vi "7-29-19 Decreasing.vi"() -> ()   [LabVIEW 2016]
uses:
  <userlib>/Levylab/LV to ITX/LVtoITX.lvclass
  <vilib>/Analysis/NI_AALPro.lvlib
panel:
  out "dG/dt Vs Temp Normalized":cluster{"Data":dbl[], "Data":dbl[]}[](graph)
  out "Slopes":cluster{dbl[], dbl[]}
  out "G Vs Time Fitted":cluster{"Data":dbl[], "Data":dbl[]}[](graph)
  out "Wavenames":string[](array[string])
  out "G Vs Time":cluster{"Data":dbl[], "Data":dbl[]}[](graph)
  out "Data":dbl[][](array[numeric])
  in  "File Path":path=path "G:/My Drive/Data/7-30 Decreasing SA03083.dat"
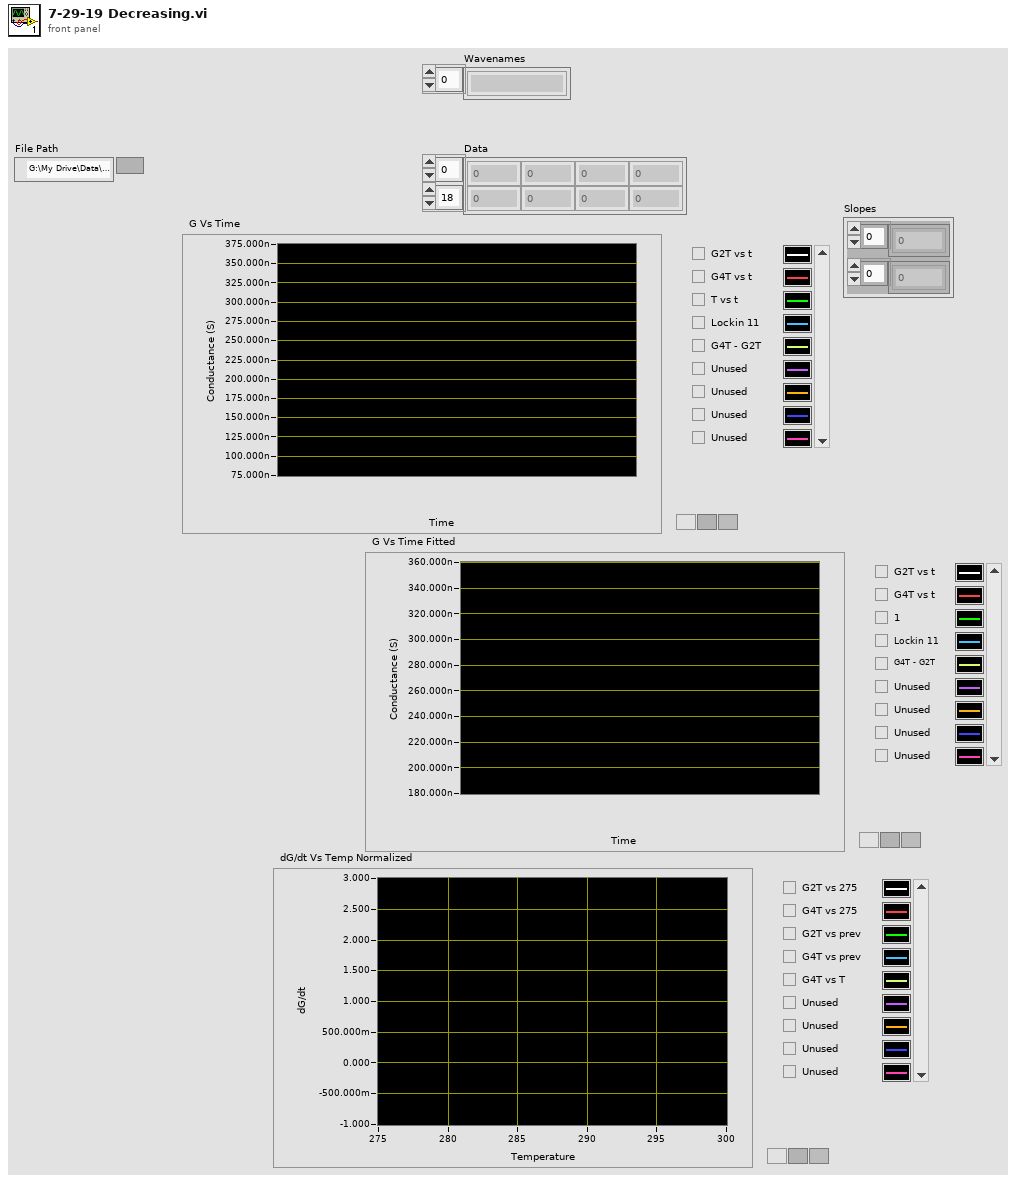
[diagram p1: front panel]
types:
  T1 = cluster{"slope min":dbl, "slope max":dbl, "intercept min":dbl, "intercept max":dbl}
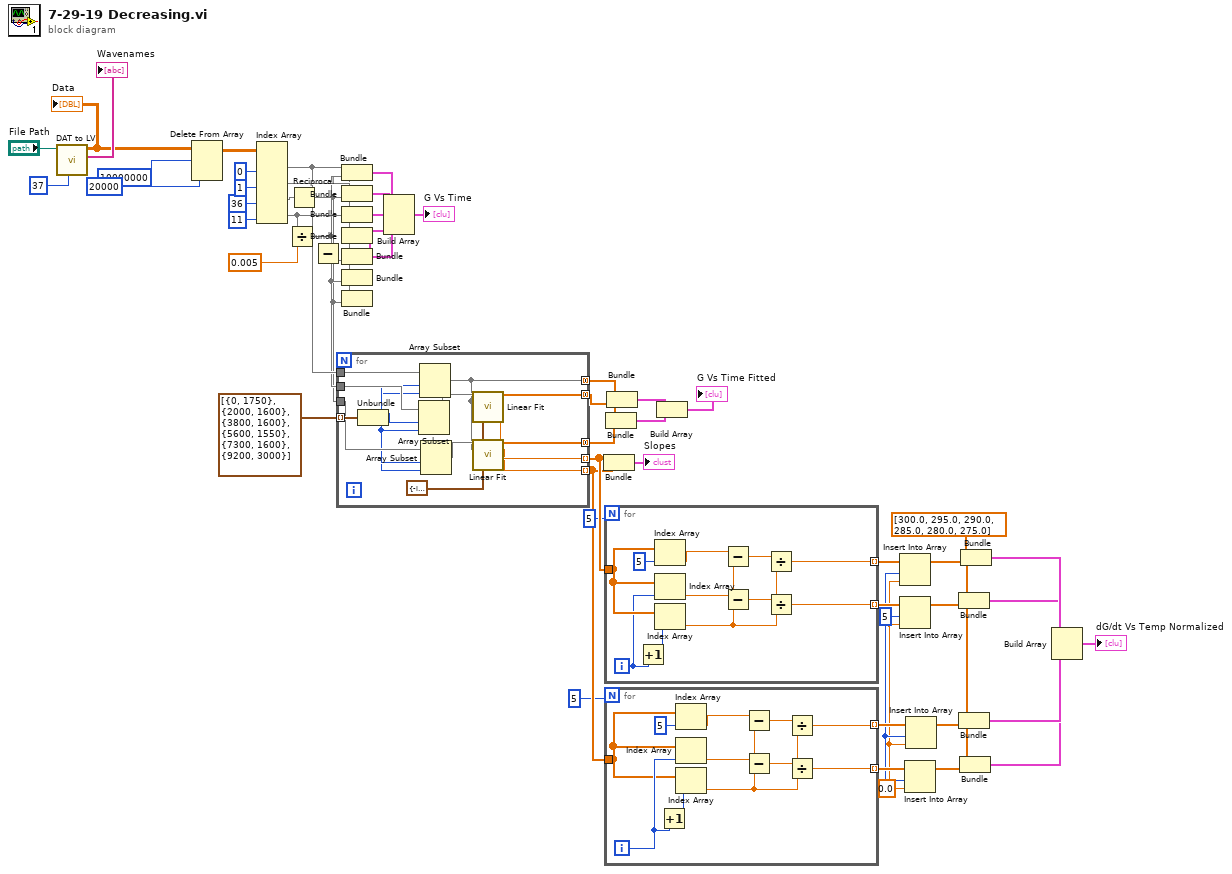
[diagram p0: block diagram]
diagram:
  w6 = dbl[] [300.0, 295.0, 290.0, 285.0, 280.0, 275.0]
  w11 = 0.0 ("new element/subarray")
  w12 = 5 ("index")
  n1 = call <userlib>:"DAT to LV.vi"("header length"=37, "File Path"="File Path") -> ("Wavenames"=→"Wavenames":string[], "Data"=w36:dbl[][])  [unwired: 6 in, 2 out]
  "Data" <- w36
  n2 = Delete From Array(array=w36, length=10000000, index (row)=20000) -> (array with subset deleted=w35:dbl[][])  [unwired: 1 in, 1 out]
  n3 = Index Array(array=w35, index (col) #1=0 ("disabled index (col)"), index (col) #2=1 ("index (col)"), index (col) #3=36 ("index (col)"), index (col) #4=11 ("index (col)")) -> (element #1=w30:dbl[], element #2=w49:dbl[], element #3=w42:dbl[], element #4=w32:dbl[])  [unwired: 4 in]
  n4 = Divide(x=w32, y=0.005) -> (x/y=w29:dbl[])
  n5 = Reciprocal(x=w42) -> (1/x=w28:dbl[])
  n6 = Subtract(x=w28, y=w29) -> (x-y=w39:dbl[])
  n7 = for {
    tunnel: cluster{"Index":i32, "Length":i32}[] [{"Index"=0, "Length"=1750}, {"Index"=2000, "Length"=1600}, {"Index"=3800, "Length"=1600}, {"Index"=5600, "Length"=1550}, {"Index"=7300, "Length"=1600}, {"Index"=9200, "Length"=3000}] -> [w67] mode=indexing
    tunnel: w30 -> [w66]
    tunnel: w29 -> [w65]
    tunnel: w28 -> [w64]
    tunnel: [w60] -> w25 mode=concatenating
    tunnel: [w59] -> w24 mode=concatenating
    tunnel: [w58] -> w20 mode=indexing
    tunnel: [w57] -> w19 mode=indexing
    tunnel: [w54] -> w26 mode=concatenating
    w61 = T1 {"slope min"=-inf, "slope max"=inf, "intercept min"=-inf, "intercept max"=inf} ("parameter bounds")
    n8 = Unbundle(w67) -> ("Index"=w63:i32, "Length"=w62:i32)
    n9 = Array Subset(array=w65, index=w63, length=w62) -> (w56:dbl[])
    n10 = Array Subset(array=w66, index=w63, length=w62) -> (w54:dbl[])
    n11 = Array Subset(array=w64, index=w63, length=w62) -> (w55:dbl[])
    n12 = call <vilib>:"Linear Fit.vi"("Y"=w56, "X"=w54, "parameter bounds"=w61) -> ("Best Linear Fit"=w60:dbl[], "slope"=w58:dbl)  [unwired: 8 in, 3 out]
    n13 = call <vilib>:"Linear Fit.vi"("Y"=w55, "X"=w54, "parameter bounds"=w61) -> ("Best Linear Fit"=w59:dbl[], "slope"=w57:dbl)  [unwired: 8 in, 3 out]
  }
  n14 = Bundle("Data"=w30, w29) -> (w34:cluster{"Data":dbl[], dbl[]})  [unwired: 1 in]
  n15 = Bundle("Data"=w30, w28) -> (w33:cluster{"Data":dbl[], dbl[]})  [unwired: 1 in]
  n16 = Bundle("Data"=w30, "Data"=w49) -> (w48:cluster{"Data":dbl[], "Data":dbl[]})  [unwired: 1 in]
  n17 = Bundle("Data"=w30, "Data"=w32) -> (w47:cluster{"Data":dbl[], "Data":dbl[]})  [unwired: 1 in]
  n18 = Bundle("Data"=w30, w39) -> (w40:cluster{"Data":dbl[], dbl[]})  [unwired: 1 in]
  n19 = Bundle("Data"=w49, w29) -> ()  [unwired: 1 in, 1 out]
  n20 = Bundle("Data"=w49, w28) -> ()  [unwired: 1 in, 1 out]
  n21 = Build Array(w34, w33, w48, w47, w40) -> (→"G Vs Time":cluster{"Data":dbl[], "Data":dbl[]}[])
  n22 = Bundle(w20, w19) -> (→"Slopes":cluster{dbl[], dbl[]})  [unwired: 1 in]
  n23 = for {
    N: 5 -> [_]
    tunnel: w20 -> [w78]
    tunnel: [w69] -> w16 mode=indexing
    tunnel: [w68] -> w15 mode=indexing
    i -> [w76]
    n24 = Increment(x=w76) -> (x+1=w77:i32)
    n25 = Index Array(array=w78, index=5) -> (element=w74:dbl)
    n26 = Index Array(array=w78, index=w76) -> (element=w73:dbl)
    n27 = Index Array(array=w78, index=w77) -> (element=w70:dbl)
    n28 = Subtract(x=w74, y=w70) -> (x-y=w72:dbl)
    n29 = Subtract(x=w73, y=w70) -> (x-y=w71:dbl)
    n30 = Divide(x=w72, y=w70) -> (x/y=w69:dbl)
    n31 = Divide(x=w71, y=w70) -> (x/y=w68:dbl)
  }
  n32 = for {
    N: 5 -> [_]
    tunnel: w19 -> [w81]
    tunnel: [w80] -> w14 mode=indexing
    tunnel: [w79] -> w13 mode=indexing
    i -> [w82]
    n33 = Increment(x=w82) -> (x+1=w83:i32)
    n34 = Index Array(array=w81, index=5) -> (element=w85:dbl)
    n35 = Index Array(array=w81, index=w82) -> (element=w86:dbl)
    n36 = Index Array(array=w81, index=w83) -> (element=w89:dbl)
    n37 = Subtract(x=w85, y=w89) -> (x-y=w87:dbl)
    n38 = Subtract(x=w86, y=w89) -> (x-y=w88:dbl)
    n39 = Divide(x=w87, y=w89) -> (x/y=w80:dbl)
    n40 = Divide(x=w88, y=w89) -> (x/y=w79:dbl)
  }
  n41 = Bundle(w26, "Best Linear Fit"=w24) -> (w23:cluster{dbl[], "Best Linear Fit":dbl[]})  [unwired: 1 in]
  n42 = Bundle(w26, "Best Linear Fit"=w25) -> (w22:cluster{dbl[], "Best Linear Fit":dbl[]})  [unwired: 1 in]
  n43 = Build Array(w22, w23) -> (→"G Vs Time Fitted":cluster{dbl[], "Best Linear Fit":dbl[]}[])
  n44 = Insert Into Array(array=w16, index=w12, new element=w11) -> (w8:dbl[])
  n45 = Insert Into Array(array=w15, index=w12, new element=w11) -> (w7:dbl[])
  n46 = Insert Into Array(array=w13, index=w12, new element=w11) -> (w9:dbl[])
  n47 = Insert Into Array(array=w14, index=w12, new element=w11) -> (w10:dbl[])
  n48 = Bundle(w6, w7) -> (w3:cluster{dbl[], dbl[]})  [unwired: 1 in]
  n49 = Bundle(w6, w10) -> (w5:cluster{dbl[], dbl[]})  [unwired: 1 in]
  n50 = Bundle(w6, w9) -> (w2:cluster{dbl[], dbl[]})  [unwired: 1 in]
  n51 = Bundle(w6, w8) -> (w4:cluster{dbl[], dbl[]})  [unwired: 1 in]
  n52 = Build Array(w4, w5, w3, w2) -> (→"dG/dt Vs Temp Normalized":cluster{dbl[], dbl[]}[])
